vi "Cargar Inventario desde archivo.vi"(8 "error in":errorcluster) -> (0 "error out":errorcluster, 3 "Productos":string[][](array[string]))   [LabVIEW 2024, in "ProductControl.lvlib"]
uses:
  ProductControl.lvlib
  <vilib>/Utility/config.llb/Read Key (String).vi
  <vilib>/Utility/config.llb/NI_LVConfig.lvlib
panel:
  # "Nombre                 Unidades                Costo Unitario"
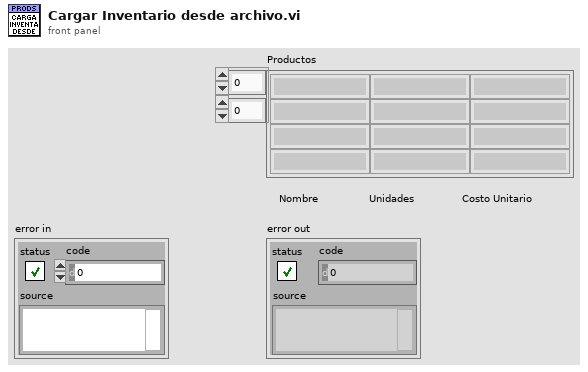
[diagram p1: front panel]
types:
  T1 = typedef "NI_LVConfig.lvlib/Config Data RefNum.ctl" = refnum<k1>
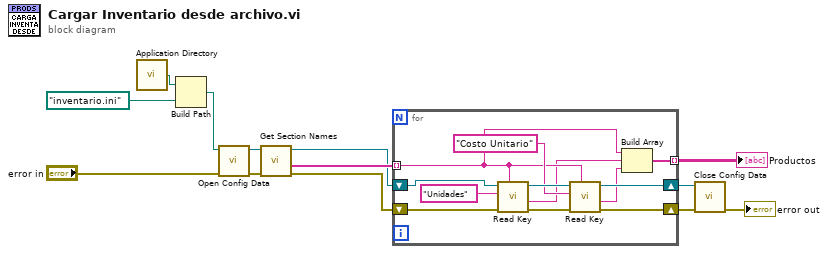
[diagram p0: block diagram]
diagram:
  n1 = call <vilib>:"Application Directory.vi"() -> ("Application Directory"=w8:path)
  n2 = Build Path(base path=w8, name or relative path=path "inventario.ini") -> (appended path=w6:path)
  n3 = call <vilib>:"Open Config Data.vi"("error in (no error)"="error in", "configuration file path"=w6) -> ("error out"=w13:errorcluster, "refnum"=w5:T1)  [unwired: 7 in, 1 out]
  n4 = call <vilib>:"Get Section Names.vi"("error in (no error)"=w13, "refnum"=w5) -> ("error out"=w12:errorcluster, "section names"=w4:string[], "refnum out"=w3:T1)  [unwired: 7 in]
  n5 = for {
    tunnel: w4 -> [w17] mode=indexing
    shift-right: [w23] -> w11
    shift-left: w12 -> [w25]
    shift-right: [w20] -> w2
    shift-left: w3 -> [w22]
    tunnel: [w14] -> w1 mode=indexing
    n6 = call-poly <vilib>:"Read Key.vi"("section"=w17, "error in (no error)"=w25, "key"="Unidades", "refnum"=w22) -> ("error out"=w24:errorcluster, "value"=w16:string, "refnum out"=w21:T1)  [unwired: 4 in, 1 out]
    n7 = call-poly <vilib>:"Read Key.vi"("section"=w17, "error in (no error)"=w24, "key"="Costo Unitario", "refnum"=w21) -> ("error out"=w23:errorcluster, "value"=w15:string, "refnum out"=w20:T1)  [unwired: 4 in, 1 out]
    n8 = Build Array(w17, w16, w15) -> (w14:string[])
  }
  "Productos" <- w1
  n9 = call <vilib>:"Close Config Data.vi"("error in (no error)"=w11, "refnum"=w2) -> ("error out"=→"error out":errorcluster)  [unwired: 8 in, 1 out]
